vi "Auto Select Close.vi"   [LabVIEW 2014]
types:
  T1 = typedef "WPI_PotentiometerDevRef.ctl" = cluster{"DevStatus":errorcluster, "Controller":T2, "Analog Channel":T3, "Invert Output":bool}
  T2 = typedef "FPGA_TypedefAnalogModule.ctl" = enum16{"Controller 1"}
  T3 = typedef "FPGA_AIChannel.ctl" = enum8{"AI 0", "AI 1", "AI 2", "AI 3", "AI MXP 0", "AI MXP 1", "AI MXP 2", "AI MXP 3", "Invalid"}
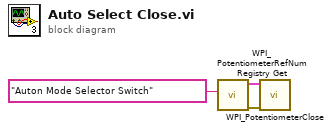
[diagram p0: block diagram]
diagram:
  n1 = call <vilib>:"WPI_PotentiometerRefNum Registry Get.vi"("refnum name"="Auton Mode Selector Switch") -> ("error out"=w1:errorcluster, "PotDevRef"=w2:T1)  [unwired: 9 in]
  n2 = call <vilib>:"WPI_PotentiometerClose.vi"("error in"=w1, "PotDevRef"=w2) -> ()  [unwired: 9 in, 1 out]
